vi "MissingIEFilesFromLVInstall.vi"() -> (2 "Code":i32, 3 "Missing IE Paths":string)   [LabVIEW 2020]
doc: "Create an 8 bit diagnostics code that is used by downstream automation.\n\nBit 0: NIIconEditor\nBit 1: lv_icon.lvlibp\nBit 2: lv_IconEditor.lvlib \nBit 3: lv_icon.vi\nBit 4: lv_icon.vit \nBit 5: SAMPLE_lv_icon.vi \nBit 6: LabVIEW Icon API \nBit 7: All non-fatal paths"
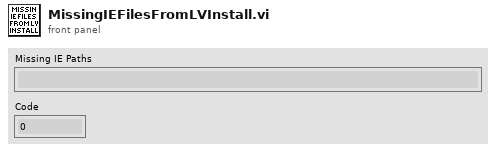
[diagram p1: front panel]
types:
  T1 = cluster{"NIIconEditor":bool, "lv_icon.lvlibp":bool, "lv_IconEditor.lvlib":bool, "lv_icon.vi":bool, "lv_icon.vit":bool, "SAMPLE_lv_icon.vi":bool, "LabVIEW Icon API":bool}
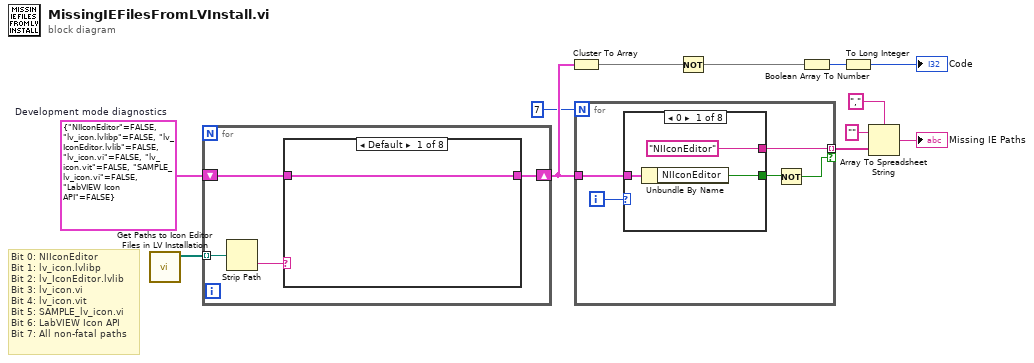
[diagram p0: block diagram]
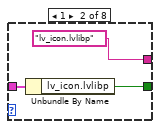
[diagram p2: hidden frame]
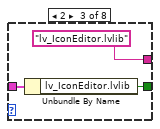
[diagram p3: hidden frame]
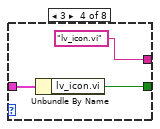
[diagram p4: hidden frame]
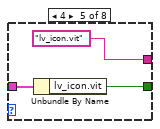
[diagram p5: hidden frame]
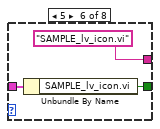
[diagram p6: hidden frame]
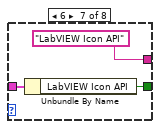
[diagram p7: hidden frame]
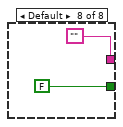
[diagram p8: hidden frame]
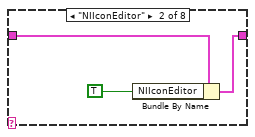
[diagram p9: hidden frame]
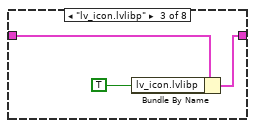
[diagram p10: hidden frame]
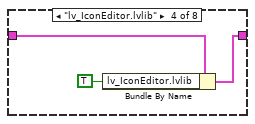
[diagram p11: hidden frame]
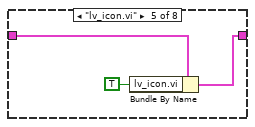
[diagram p12: hidden frame]
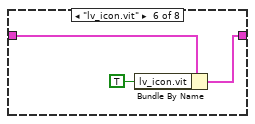
[diagram p13: hidden frame]
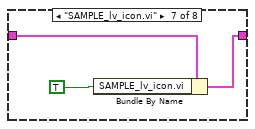
[diagram p14: hidden frame]
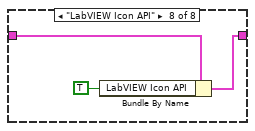
[diagram p15: hidden frame]
diagram:
  w11 = T1 {"NIIconEditor"=FALSE, "lv_icon.lvlibp"=FALSE, "lv_IconEditor.lvlib"=FALSE, "lv_icon.vi"=FALSE, "lv_icon.vit"=FALSE, "SAMPLE_lv_icon.vi"=FALSE, "LabVIEW Icon API"=FALSE}  # Development mode diagnostics
  # "Bit 0: NIIconEditor\nBit 1: lv_icon.lvlibp\nBit 2: lv_IconEditor.lvlib \nBit 3: lv_icon.vi\nBit 4: lv_icon.vit \nBit 5: SAMPLE_lv_icon.vi \nBit 6: LabVIEW Icon API \nBit 7: All non-fatal paths"
  n1 = call "Get Paths to Icon Editor Files in LV Installation.vi"() -> ("absolute paths"=w12:path[])  [unwired: 10 in, 1 out]
  n2 = for {
    tunnel: w12 -> [w13] mode=indexing
    shift-right: [w14] -> w4
    shift-left: w11 -> [w15]
    n3 = Strip Path(path=w13) -> (name=w16:string)  [unwired: 1 out]
    n4 = case shown="Default" w16 {
      tunnel: w15 -> [w17 w20 w23 w26 w29 w32 w35 w38]
      tunnel: [w17 w19 w22 w25 w28 w31 w34 w37] -> w14
      frame Default {
      }
      frame "NIIconEditor" {
        n5 = Bundle By Name(cluster=w20, "NIIconEditor"=TRUE) -> (w19:T1)
      }
      frame "lv_icon.lvlibp" {
        n6 = Bundle By Name(cluster=w23, "lv_icon.lvlibp"=TRUE) -> (w22:T1)
      }
      frame "lv_IconEditor.lvlib" {
        n7 = Bundle By Name(cluster=w26, "lv_IconEditor.lvlib"=TRUE) -> (w25:T1)
      }
      frame "lv_icon.vi" {
        n8 = Bundle By Name(cluster=w29, "lv_icon.vi"=TRUE) -> (w28:T1)
      }
      frame "lv_icon.vit" {
        n9 = Bundle By Name(cluster=w32, "lv_icon.vit"=TRUE) -> (w31:T1)
      }
      frame "SAMPLE_lv_icon.vi" {
        n10 = Bundle By Name(cluster=w35, "SAMPLE_lv_icon.vi"=TRUE ("lv_icon.vit")) -> (w34:T1)
      }
      frame "LabVIEW Icon API" {
        n11 = Bundle By Name(cluster=w38, "LabVIEW Icon API"=TRUE) -> (w37:T1)
      }
    }
  }
  n12 = Cluster To Array(cluster=w4) -> (array=w3:bool[])
  n13 = for {
    N: 7 -> [_]
    tunnel: w4 -> [w42]
    tunnel: [w41] -> w10 mode=indexing if=w40
    i -> [w43]
    n14 = case shown="0" w43 {
      tunnel: w42 -> [w46 w49 w52 w55 w58 w61 w64 _]
      tunnel: ["NIIconEditor" "lv_icon.lvlibp" "lv_IconEditor.lvlib" "lv_icon.vi" "lv_icon.vit" "SAMPLE_lv_icon.vi" "LabVIEW Icon API" ""] -> w41
      tunnel: [w44 w47 w50 w54 w56 w59 w62 FALSE ("NIIconEditor")] -> w39
      frame 0 {
        n15 = Unbundle By Name(w46) -> ("NIIconEditor"=w44:bool)
      }
      frame 1 {
        n16 = Unbundle By Name(w49) -> ("lv_icon.lvlibp"=w47:bool)
      }
      frame 2 {
        n17 = Unbundle By Name(w52) -> ("lv_IconEditor.lvlib"=w50:bool)
      }
      frame 3 {
        n18 = Unbundle By Name(w55) -> ("lv_icon.vi"=w54:bool)
      }
      frame 4 {
        n19 = Unbundle By Name(w58) -> ("lv_icon.vit"=w56:bool)
      }
      frame 5 {
        n20 = Unbundle By Name(w61) -> ("SAMPLE_lv_icon.vi"=w59:bool)
      }
      frame 6 {
        n21 = Unbundle By Name(w64) -> ("LabVIEW Icon API"=w62:bool)
      }
      frame Default {
      }
    }
    n22 = Not(x=w39) -> (.not. x?=w40:bool)
  }
  n23 = Not(x=w3) -> (.not. x?=w2:bool[])
  n24 = Boolean Array To Number(Boolean array=w2) -> (number=w6:u32)
  n25 = To Long Integer(number=w6) -> (32bit integer=→"Code":i32)
  n26 = Array To Spreadsheet String(delimiter (Tab)=",", array=w10, 3:"" ("format string")) -> (spreadsheet string=→"Missing IE Paths":string)
